vi "Test_Chan_1.vi"(7 "Signal I/O_Clk":refnum<k21>="Mezza_DIO/DIO16", 8 "Enable_ON":bool, 9 "Stop":bool, 10 "Enable_RE":bool, 11 "Signal I/O":refnum<k21>="Mezza_DIO/DIO2") -> (1 "Clk":bool, 3 "Signal":bool)   [LabVIEW 2011]
uses:
  <vilib>/rvi/eio/common/nirviEmuTemplateMethod_errors.vi
  <vilib>/eio/EIONode/EIONode.xnode
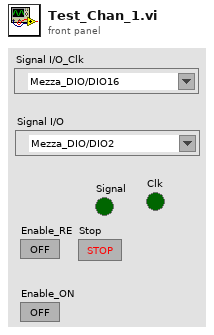
[diagram p1: front panel]
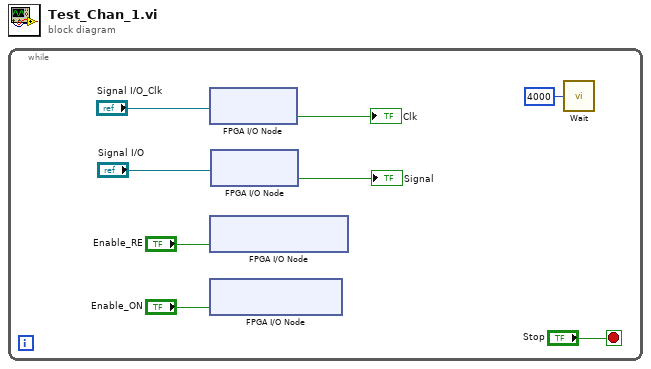
[diagram p0: block diagram]
diagram:
  n1 = while {
    stop <- "Stop" stop-if-true
    n2 = xnode "FPGA I/O Node"("FPGA I/O In"="Signal I/O_Clk") -> ("I/O Item"=→"Clk":bool)  [unwired: 1 out]
    n3 = xnode "FPGA I/O Node"("Mezza_DIO/DIO32"="Enable_RE") -> ()  [unwired: 1 in, 1 out]
    n4 = xnode "FPGA I/O Node"("Mezza_DIO/DIO0"="Enable_ON") -> ()  [unwired: 1 in, 1 out]
    n5 = xnode "FPGA I/O Node"("FPGA I/O In"="Signal I/O") -> ("I/O Item"=→"Signal":bool)  [unwired: 1 out]
    n6 = call "Wait"("Count(Ticks)"=u32 4000) -> ()  [unwired: 1 out]
  }
